vi "InitMouse.vi"(2 "Mouse States":T1[](array[typedef]), 8 "error in (no error)":errorcluster, 11 "Input in":refnum<class "Input.lvclass">) -> (0 "error out":errorcluster, 3 "Input out":refnum<class "Input.lvclass">)   [LabVIEW 2009, in "Input.lvclass"]
uses:
  Input.lvclass
  Mouse State.ctl
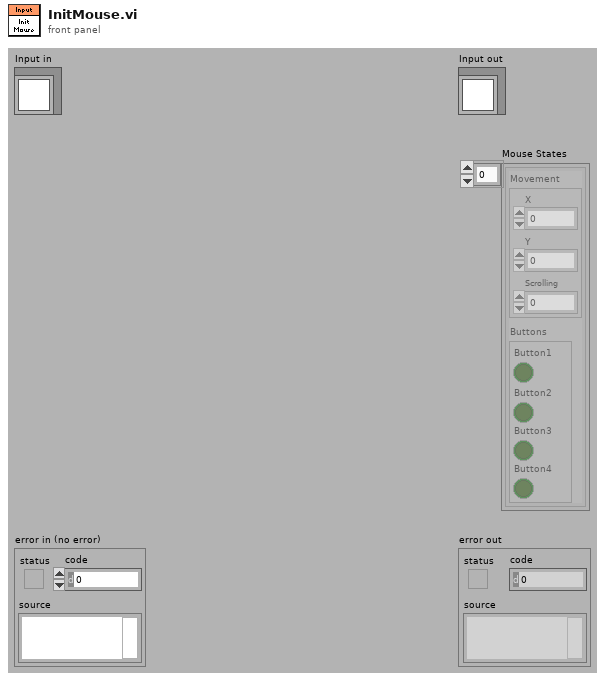
[diagram p1: front panel]
types:
  T1 = typedef "Input.lvclass/Mouse State.ctl" = cluster{"Movement":cluster{"X":i32, "Y":i32, "Scrolling":i32}, "Buttons":cluster{"Button1":bool, "Button2":bool, "Button3":bool, "Button4":bool}}
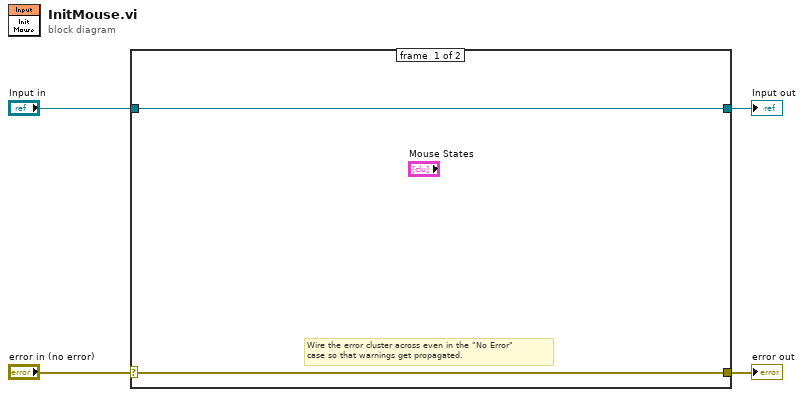
[diagram p0: block diagram]
diagram:
  n1 = case shown="No Error" "error in (no error)" {
    selector: "error in (no error)" -> [w5 w8]
    tunnel: [w5 w8] -> w3
    tunnel: [w6 w7] -> w1
    tunnel: "Input in" -> [w6 w7]
    frame #0 {
      # "Wire the error cluster across even in the \"No Error\"\ncase so that warnings get propagated."
    }
    frame #1 {
    }
  }
  "error out" <- w3
  "Input out" <- w1
